vi "CRM error handler.vi"(8 "Error In":errorcluster) -> (0 "Error Out":errorcluster, 2 "Exit?":bool)   [LabVIEW 2016]
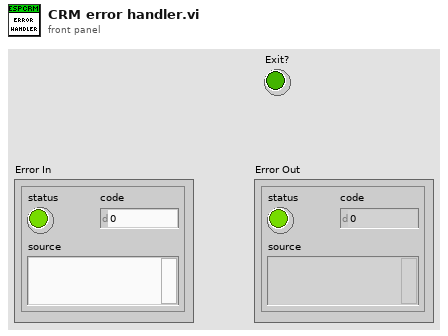
[diagram p1: front panel]
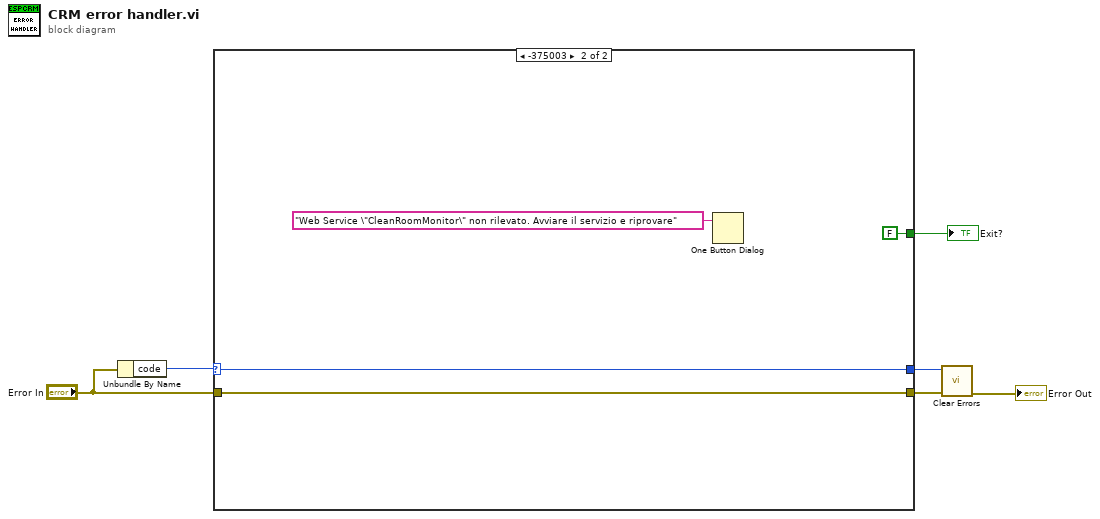
[diagram p0: block diagram]
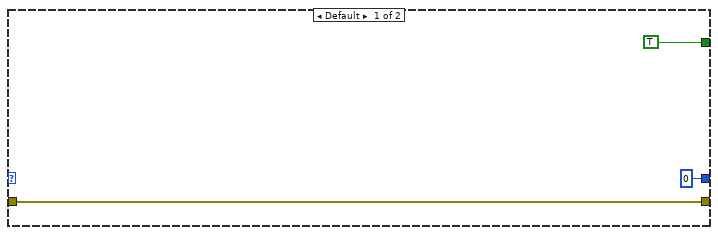
[diagram p2: hidden frame]
diagram:
  n1 = Unbundle By Name("Error In") -> ("code"=w6:i32)
  n2 = case shown="-375003" w6 {
    selector: w6 -> [_ w12]
    tunnel: "Error In" -> [w8 w13]
    tunnel: [w8 w13] -> w4
    tunnel: [0 ("code") w12] -> w2
    tunnel: [TRUE FALSE] -> w1
    frame Default {
    }
    frame -375003 {
      n3 = One Button Dialog(message="Web Service \"CleanRoomMonitor\" non rilevato. Avviare il servizio e riprovare") -> ()  [unwired: 1 in, 1 out]
    }
  }
  "Exit?" <- w1
  n4 = call <vilib>:"Clear Errors.vi"("error in (no error)"=w4, "specific error code to clear (0: all)"=w2) -> ("error out"=→"Error Out":errorcluster)  [unwired: 4 in, 1 out]
